vi "ReadWrite.vi"(8 "error in (no error)":errorcluster, 11 "Node Ptr":T2 format="%.0x") -> (0 "error out":errorcluster)   [LabVIEW 2017, in "Shared Variables CD 2.0 Configuration.lvlib"]
uses:
  Shared Variables CD 2.0 Configuration.lvlib
  <vilib>/NI Veristand/Custom Device API/Custom Device Item Ref.ctl
  Support/Add SV Process/Channel Configuration States.ctl
  Support/ChannelVS/ChannelVS.lvclass
  C:/Users/Public/Documents/National Instruments/NI VeriStand 2017/Custom Devices/Shared Variables CD 2.0/Data/Channel.lvlibp/Channel.lvclass
  <vilib>/Utility/VariantDataType/Type.ctl
  Support/ChannelVS/ChannelVS.lvclass/ChannelVS.ctl
  Support/ChannelVS/Compare Ch with Ch List.vi
  Support/ChannelVS/Read VeriSTAND Channel Info.vi
  Support/ChannelVS/Write VeriSTAND Channel Info.vi
  Shared/SV Global.vi
  Public/Documents/National Instruments/NI VeriStand 2017/Custom Devices/Shared Variables CD 2.0/Data/Channel.lvlibp/Read Channel Info.vi
  <vilib>/NI VeriStand/Custom Device API/Custom Device API.lvlib
  <vilib>/Utility/VariantDataType/VariantType.lvlib
panel:
  out "State":T1
  in  "Remove Button":bool
  in  "Add Button":bool
  in  "Refresh Target":bool
  in  "Target IPAddr":string caption="Target IP Address*"
  in  "Target List":string[](tree)
  in  "CD List":string[](tree)
  in  "Header":cluster{"Section Name":string}={"Section Name"="Custom Device Item Settings"}
  in  "Description":string
  in  "Name":string
  # "*Do Not Use \"localhost\" or host name"
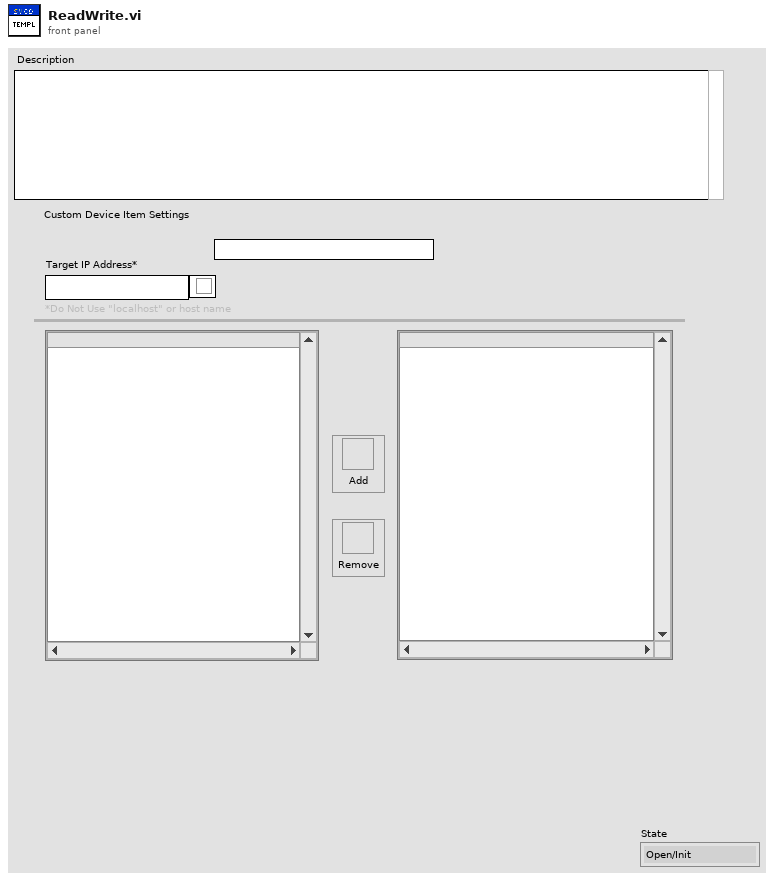
[diagram p1: front panel]
types:
  T1 = typedef "Shared Variables CD 2.0 Configuration.lvlib/Channel Configuration States.ctl" = enum16{"Open/Init", "Start Update", "Get VS Channels", "Get Available Ch from Target", "Wait On User Action", "Update Target Tree", "Update VS Trees", "Update Done", "Create VS Channels", "Remove VS Channels", "Error", "Close"}
  T2 = typedef "Custom Device API.lvlib/Custom Device Item Ref.ctl" = u64
  T3 = cluster{"Read Channel Array":refnum<class "ChannelVS.lvclass">[], "Write Channel Array":refnum<class "ChannelVS.lvclass">[]}
  T4 = enum8{"Enabled", "Disabled", "Disabled and Grayed Out"}
  T5 = typedef "VariantType.lvlib/Type.ctl" = enum8{"Invalid Type", "Void", "I8", "I16", "I32", "I64", "U8", "U16", "U32", "U64", "Single Float", "Double Float", "Extended Float", "Single Complex", "Double Complex", "Extended Complex", "Enum U8", "Enum U16", "Enum U32", "Enum U64", "Single Float With Unit", "Double Float With Unit", "Extended Float With Unit", "Single Complex with Unit", "Double Complex with Unit", "Extended Complex with Unit", "Boolean", "String", "Path", "Picture", "Tag", "Array", "Cluster", "Variant", "LV Variant", "Waveform", "Timestamp", "Digital Waveform", "Digital Data", "ExpressData", "Refnum", "External Data", "VI", "Poly VI", "LabVIEW Class Instance", "Fixed Point"}
  T6 = typedef "Custom Device API.lvlib/Custom Device Item Info.ctl" = cluster{"Name":string, "Is Channel":bool, "GUID":string, "Is Waveform":bool}
  T7 = typedef "Custom Device API.lvlib/Custom Device Commands.ctl" = enum16{"Default", "Item renamed", "Shutdown", "Dynamic button pressed"}
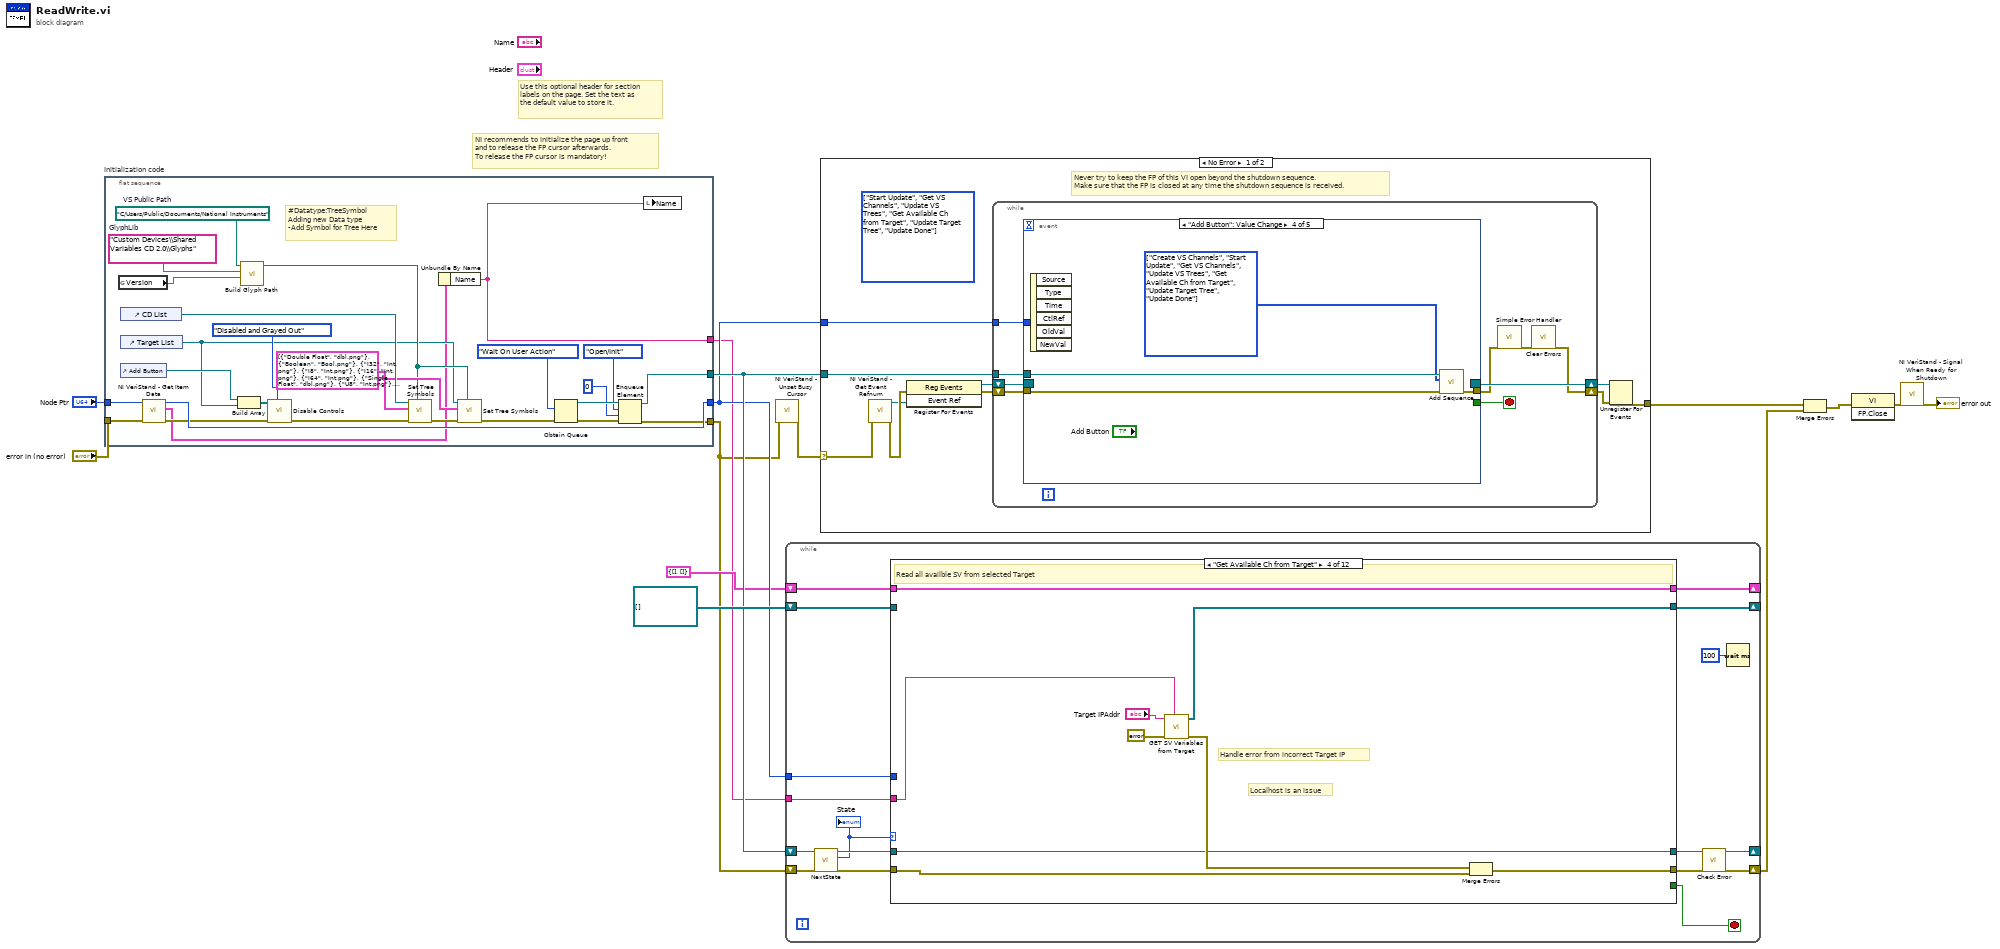
[diagram p0: block diagram]
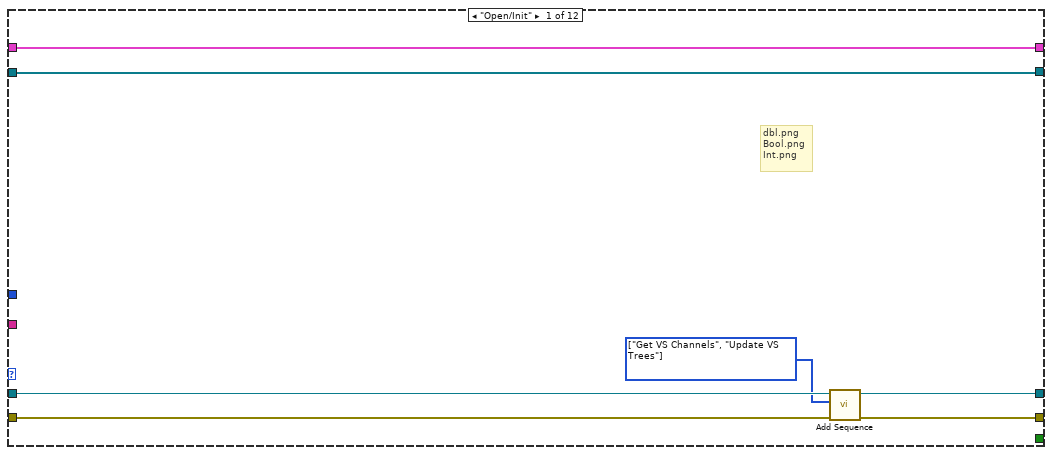
[diagram p2: hidden frame]
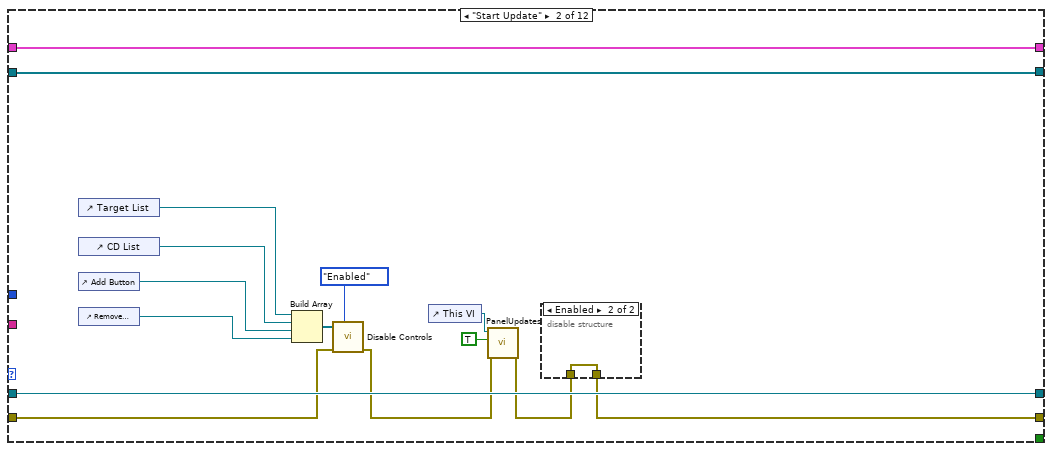
[diagram p3: hidden frame]
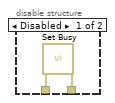
[diagram p4: hidden frame]
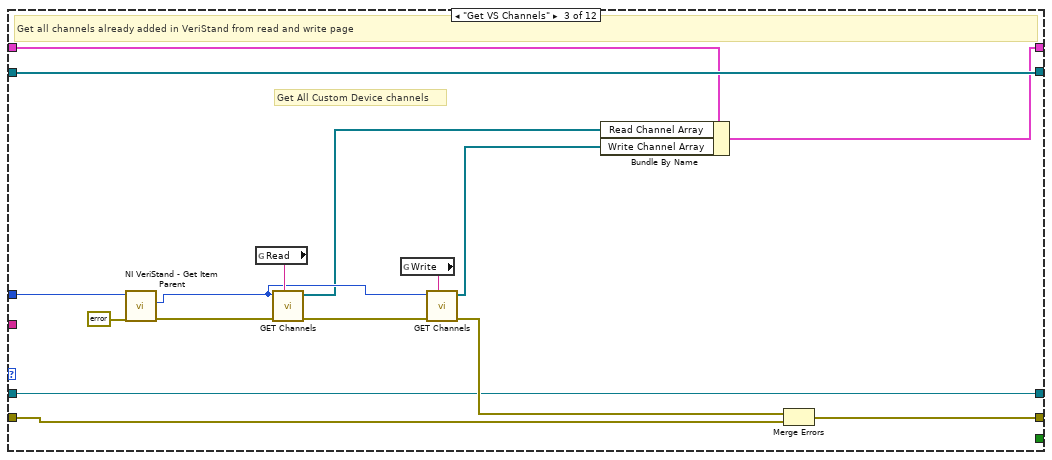
[diagram p5: hidden frame]
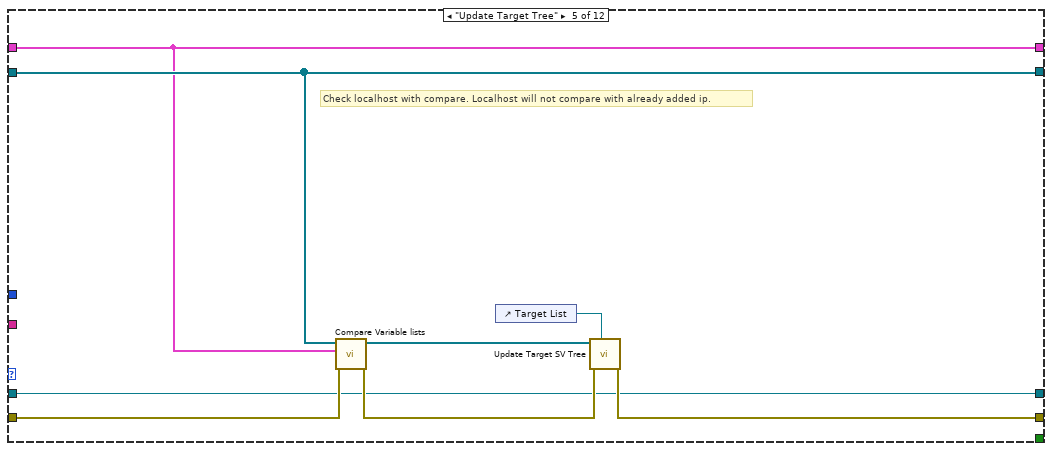
[diagram p6: hidden frame]
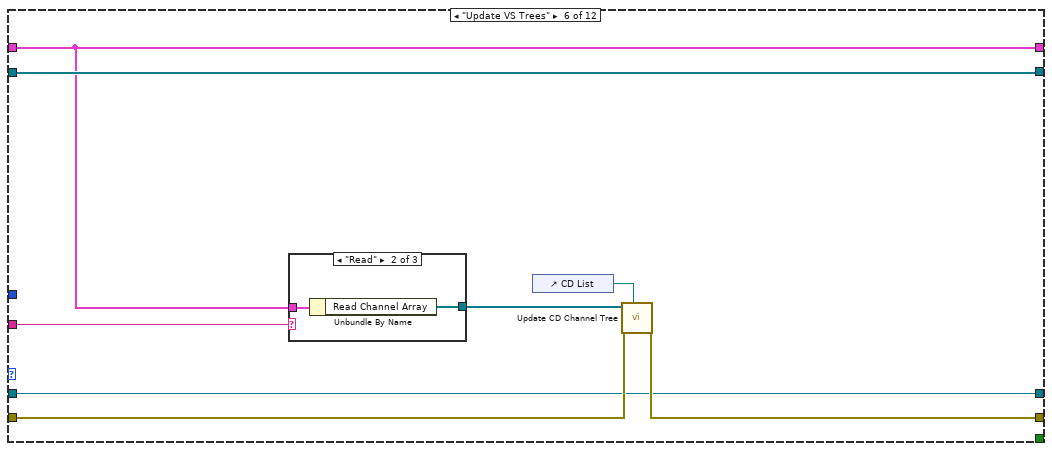
[diagram p7: hidden frame]
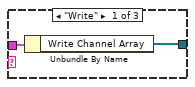
[diagram p8: hidden frame]
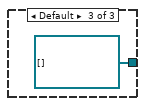
[diagram p9: hidden frame]
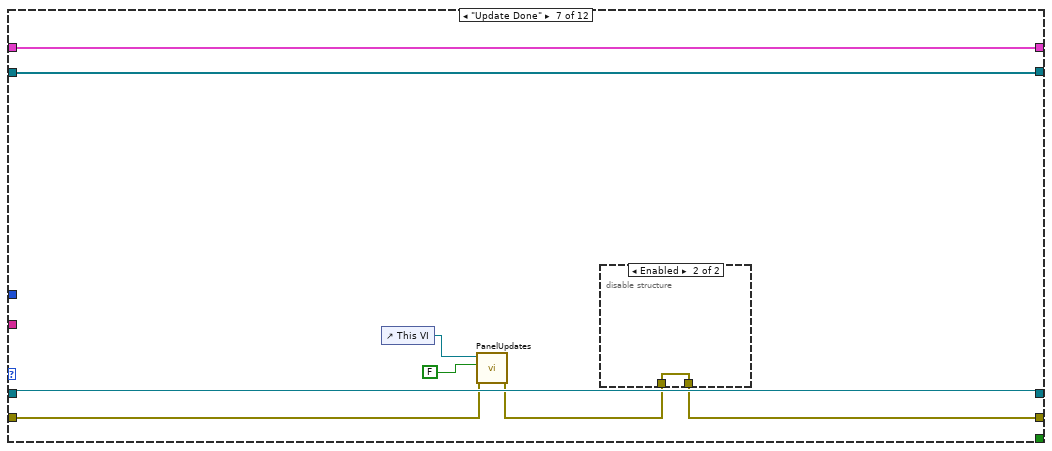
[diagram p10: hidden frame]
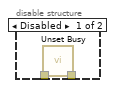
[diagram p11: hidden frame]
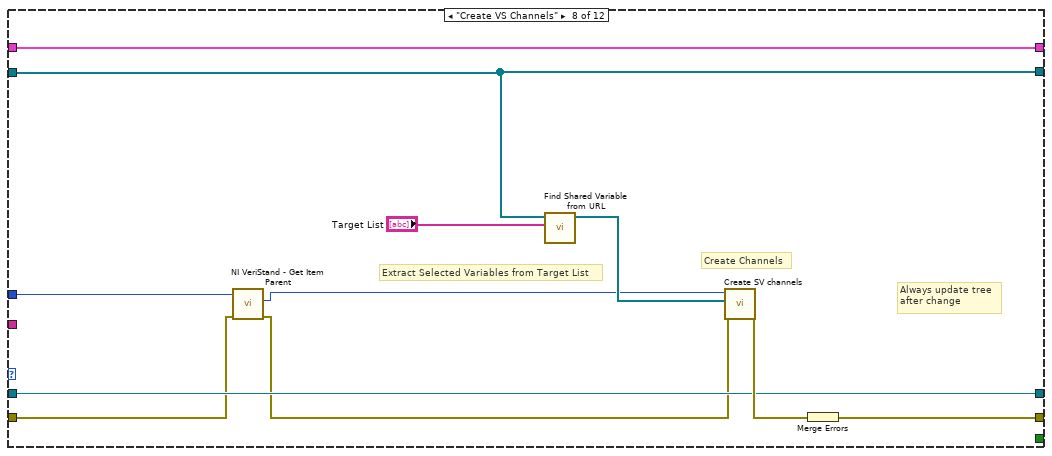
[diagram p12: hidden frame]
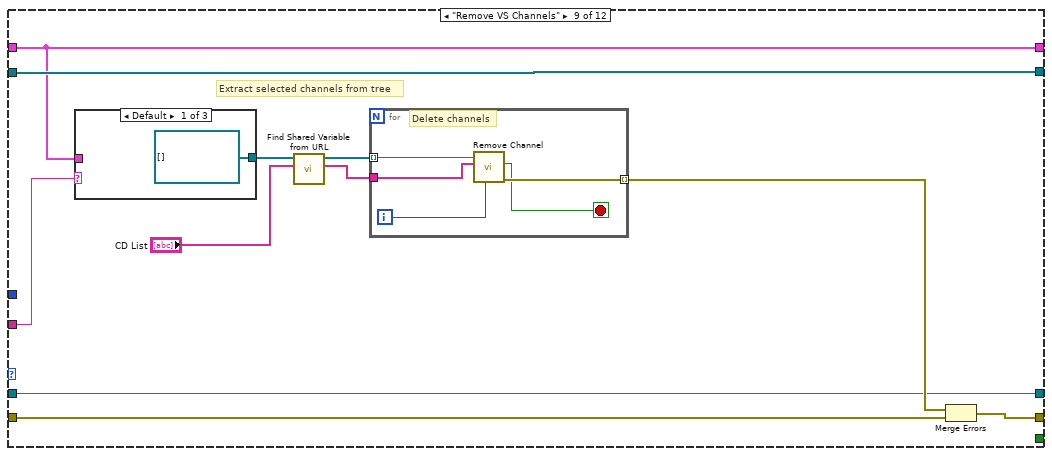
[diagram p13: hidden frame]
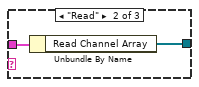
[diagram p14: hidden frame]
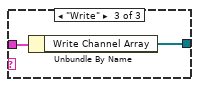
[diagram p15: hidden frame]
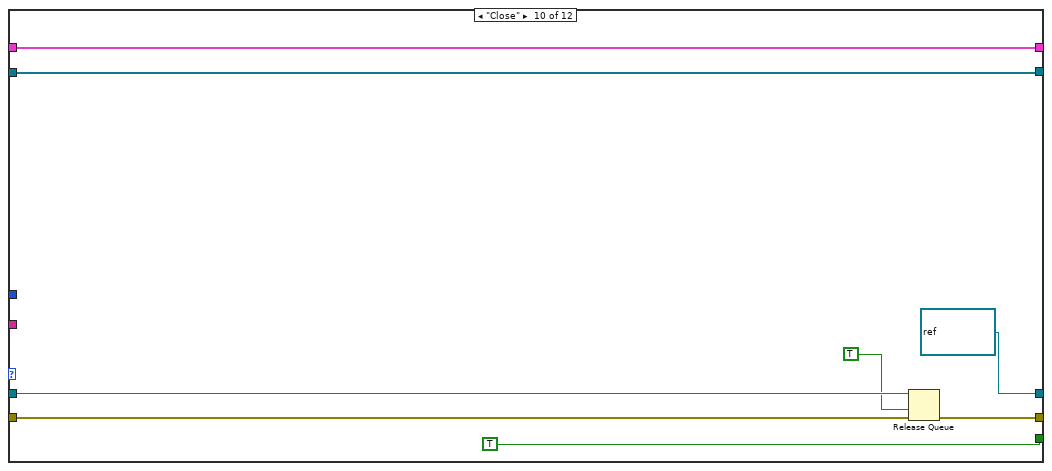
[diagram p16: hidden frame]
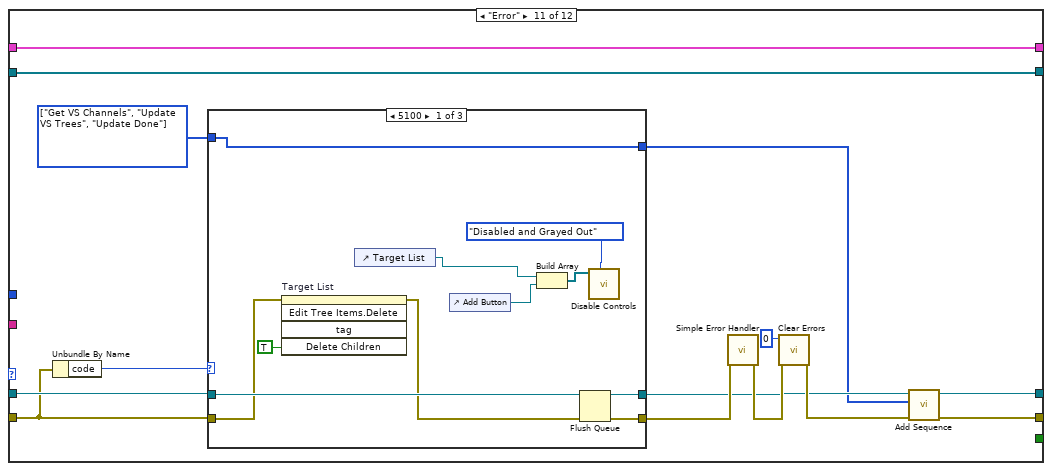
[diagram p17: hidden frame]
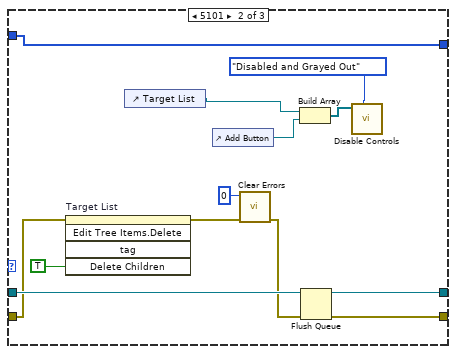
[diagram p18: hidden frame]
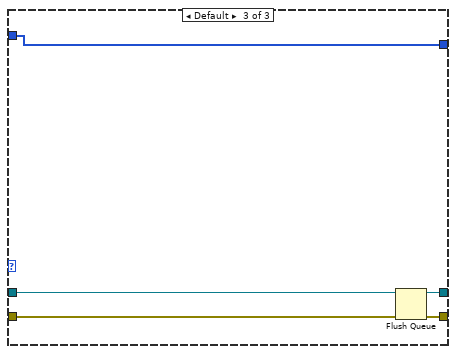
[diagram p19: hidden frame]
diagram:
  # "Use this optional header for section labels on the page. Set the text as the default value to store it."
  # "NI recommends to initialize the page up front\nand to release the FP cursor afterwards.\nTo release the FP cursor is mandatory!"
  n1 = flat-sequence "Initialization code" {
    tunnel: "error in (no error)" -> [w38]
    tunnel: "Node Ptr" -> [w39]
    tunnel: [w40] -> w6
    tunnel: [w25] -> w1
    tunnel: [w24] -> w7
    tunnel: [w15] -> w4
    frame #0 {
      w36 = path "C:/Users/Public/Documents/National Instruments"  # VS Public Path
      w37 = "Custom Devices\\Shared Variables CD 2.0\\Glyphs"  # GlyphLib
      w32 = cluster{"Type":T5, string}[] [{"Type"=enum."Double Float", "dbl.png"}, {"Type"=enum."Boolean", "Bool.png"}, {"Type"=enum."I32", "Int.png"}, {"Type"=enum."I8", "Int.png"}, {"Type"=enum."I16", "Int.png"}, {"Type"=enum."I64", "Int.png"}, {"Type"=enum."Single Float", "dbl.png"}, {"Type"=enum."U8", "Int.png"}, {"Type"=enum."U16", "Int.png"}, {"Type"=enum."U32", "Int.png"}, {"Type"=enum."U64", "Int.png"}]
      # "#Datatype:TreeSymbol\nAdding new Data type\n-Add Symbol for Tree Here"
      n2 = global read "SV Global.vi" "Version"() -> (w35:string)
      n3 = control-ref of="CD List"() -> (w34:refnum<vi>)
      n4 = control-ref of="Add Button"() -> (w22:refnum<vi>)
      n5 = control-ref of="Target List"() -> (w18:refnum<vi>)
      n6 = call <vilib>:"NI VeriStand - Get Item Data.vi"("error in (no error)"=w38, "Item Ref in"=w39) -> ("error out"=w20:errorcluster, "Item Info"=w16:T6, "Item Ref out"=w40:T2)  [unwired: 6 in, 1 out]
      n7 = Build Array(w22, w18) -> (w23:refnum<vi>[])
      n8 = call "Build Glyph Path.vi"("Version"=w35, "GlyphLib"=w37, "VS Public Path"=w36) -> ("Path to Glyph Lib"=w31:path)  [unwired: 8 in]
      n9 = call "Disable Controls.vi"("Disabled"=T4."Disabled and Grayed Out", "error in (no error)"=w20, "Array"=w23) -> ("error out"=w19:errorcluster)  [unwired: 8 in]
      n10 = call "Set Tree Symbols.vi"("Path to PNG lib"=w31, "error in (no error)"=w19, "Index and Image"=w32, "TreeControl in"=w34) -> ("error out"=w33:errorcluster)  [unwired: 7 in]
      n11 = Unbundle By Name(w16) -> ("Name"=w15:string)
      n12 = call "Set Tree Symbols.vi"("Path to PNG lib"=w31, "error in (no error)"=w33, "Index and Image"=w32, "TreeControl in"=w18) -> ("error out"=w17:errorcluster)  [unwired: 7 in]
      n13 = Obtain Queue(element data type=Channel_Configuration_States."Wait On User Action", error in (no error)=w17) -> (queue out=w30:refnum<queue>, error out=w29:errorcluster)  [unwired: 3 in, 1 out]
      n14 = Enqueue Element(queue=w30, element=Channel_Configuration_States."Open/Init", timeout in ms (-1)=0, error in (no error)=w29) -> (queue out=w24:refnum<queue>, error out=w25:errorcluster)  [unwired: 1 out]
      n15 = local write "Name"(w15) -> ()
    }
  }
  n16 = call <vilib>:"NI VeriStand - Unset Busy Cursor.vi"("error in (no error)"=w1) -> ("error out"=w10:errorcluster)  [unwired: 10 out]
  n17 = while {
    shift-right: [w50] -> w2
    shift-left: w1 -> [w43]
    shift-right: [w57] -> _
    shift-left: T3 {"Read Channel Array"=[], "Write Channel Array"=[]} -> [w56]
    shift-right: [w54] -> _
    shift-left: refnum<class "ChannelVS.lvclass">[] [] ("Channel Array") -> [w53]
    shift-right: [w45] -> _
    shift-left: w7 -> [w49]
    tunnel: w6 -> [w42]
    tunnel: w4 -> [w41]
    stop <- w55 stop-if-true
    n18 = call "NextState.vi"("error in (no error)"=w43, "Queue in"=w49) -> ("error out"=w44:errorcluster, "Next State"=w47:T1, "Queue out"=w48:refnum<queue>)  [unwired: 7 in]
    "State" <- w47
    n19 = case shown="\"Get Available Ch from Target\"" w47 {
      tunnel: w44 -> [w58 w67 w95 w103 w113 w121 w133 w145 w161 w176 w189 w226]
      tunnel: [w60 w68 w96 w104 w115 w120 w129 w148 w158 w175 w183 w226] -> w51
      tunnel: [w64 w79 w84 w107 w109 w122 w136 w150 w159 w178 w193 w225] -> w57
      tunnel: w56 -> [w64 w79 w83 w107 w109 w122 w136 w150 w159 w178 w193 w225]
      tunnel: [_ _ _ _ _ _ _ _ _ TRUE _ _] -> w55
      tunnel: [w63 w78 w98 w101 w111 w123 w135 w142 w160 w177 w192 w224] -> w54
      tunnel: w53 -> [w63 w78 w98 _ w111 w123 w135 w142 w160 w177 w192 w224]
      tunnel: w48 -> [w62 w72 w93 w102 w112 w119 w134 w147 w156 w174 w190 w223]
      tunnel: [w61 w72 w93 w102 w112 w119 w134 w147 w156 w172 w181 w223] -> w46
      tunnel: w42 -> [_ _ w85 _ _ _ _ w140 _ _ _ _]
      tunnel: w41 -> [_ _ _ w99 _ w116 _ _ w151 _ _ _]
      frame "Open/Init" {
        w59 = T1[] [enum."Get VS Channels", enum."Update VS Trees"] items=["Open/Init", "Start Update", "Get VS Channels", "Get Available Ch from Target", "Wait On User Action", "Update Target Tree", "Update VS Trees", "Update Done", "Create VS Channels", "Remove VS Channels", "Error", "Close"]
        # "dbl.png\nBool.png\nInt.png"
        n20 = call "Add Sequence.vi"("error in (no error)"=w58, "Transition Sequence"=w59, "Queue in"=w62) -> ("error out"=w60:errorcluster, "Queue out"=w61:refnum<queue>)  [unwired: 7 in]
      }
      frame "Start Update" {
        n21 = control-ref of="Target List"() -> (w65:refnum<vi>)
        n22 = control-ref of="CD List"() -> (w76:refnum<vi>)
        n23 = control-ref of="Add Button"() -> (w77:refnum<vi>)
        n24 = control-ref of="Remove Button"() -> (w74:refnum<vi>)
        n25 = Build Array(w65, w76, w77, w74) -> (w73:refnum<vi>[])
        n26 = call "Disable Controls.vi"("Disabled"=T4."Enabled", "error in (no error)"=w67, "Array"=w73) -> ("error out"=w66:errorcluster)  [unwired: 8 in]
        n27 = control-ref of="This VI"() -> (w70:refnum<vi>)
        n28 = call "PanelUpdates.vi"("error in (no error)"=w66, "Defer Panel Updates"=TRUE, "VI in"=w70) -> ("error out"=w69:errorcluster)  [unwired: 8 in]
        n29 = disable-structure shown="Enabled" {
          disable-tunnel: w69 -> [w81 w82]
          disable-tunnel: [w80 w82] -> w68
          frame Disabled {
            n30 = call <vilib>:"Set Busy.vi"("error in (no error)"=w81) -> ("error out"=w80:errorcluster)  [unwired: 9 in, 1 out]
          }
          frame Enabled {
          }
        }
      }
      frame "Get VS Channels" {
        # "Get All Custom Device channels"
        # "Get all channels already added in VeriStand from read and write page"
        n31 = call <vilib>:"NI VeriStand - Get Item Parent.vi"("error in (no error)"=errorcluster {"status"=FALSE, "code"=0, "source"=""}, "Item Ref in"=w85) -> ("error out"=w90:errorcluster, "Parent Ref"=w88:T2)  [unwired: 6 in, 2 out]
        n32 = global read "SV Global.vi" "Read"() -> (w91:string)
        n33 = call "GET Channels.vi"("Channel Direction"=w91, "error in (no error)"=w90, "Item Ref in"=w88) -> ("error out"=w89:errorcluster, "VS Channel Array"=w87:refnum<class "ChannelVS.lvclass">[])  [unwired: 7 in]
        n34 = global read "SV Global.vi" "Write"() -> (w92:string)
        n35 = call "GET Channels.vi"("Channel Direction"=w92, "error in (no error)"=w89, "Item Ref in"=w88) -> ("error out"=w97:errorcluster, "VS Channel Array"=w86:refnum<class "ChannelVS.lvclass">[])  [unwired: 7 in]
        n36 = Bundle By Name(cluster=w83, "Read Channel Array"=w87, "Write Channel Array"=w86) -> (w84:T3)
        n37 = Merge Errors(w97, w95) -> (w96:errorcluster)
      }
      frame "Get Available Ch from Target" {
        # "Localhost is an issue"
        # "Handle error from incorrect Target IP"
        # "Read all availble SV from selected Target"
        n38 = call "GET SV Variables from Target.vi"("Read/Write"=w99, "error in (no error)"=errorcluster {"status"=FALSE, "code"=0, "source"=""}, "Target"="Target IPAddr") -> ("error out"=w106:errorcluster, "Channel Array"=w101:refnum<class "ChannelVS.lvclass">[])  [unwired: 7 in]
        n39 = Merge Errors(w106, w103) -> (w104:errorcluster)
      }
      frame "Update Target Tree" {
        # "Check localhost with compare. Localhost will not compare with already added ip."
        n40 = call "Compare Variable lists.vi"("error in (no error)"=w113, "Channel Arrays"=w109, "Variable List"=w111) -> ("error out"=w114:errorcluster, "Variable list compared"=w110:refnum<class "ChannelVS.lvclass">[])  [unwired: 7 in]
        n41 = control-ref of="Target List"() -> (w108:refnum<vi>)
        n42 = call "Update Target SV Tree.vi"("TreeControl in"=w108, "error in (no error)"=w114, "Variable list compared"=w110) -> ("error out"=w115:errorcluster)  [unwired: 8 in]
      }
      frame "Update VS Trees" {
        n43 = case shown="\"Read\"" w116 {
          tunnel: [w125 w127 refnum<class "ChannelVS.lvclass">[] [] ("Read Channel Array")] -> w118
          tunnel: w122 -> [w124 w126 _]
          frame "Write" {
            n44 = Unbundle By Name(w124) -> ("Write Channel Array"=w125:refnum<class "ChannelVS.lvclass">[])
          }
          frame "Read" {
            n45 = Unbundle By Name(w126) -> ("Read Channel Array"=w127:refnum<class "ChannelVS.lvclass">[])
          }
          frame Default {
          }
        }
        n46 = control-ref of="CD List"() -> (w117:refnum<vi>)
        n47 = call "Update CD Channel Tree.vi"("CD List"=w117, "error in (no error)"=w121, "Channel Array"=w118) -> ("error out"=w120:errorcluster)  [unwired: 8 in]
      }
      frame "Update Done" {
        n48 = control-ref of="This VI"() -> (w132:refnum<vi>)
        n49 = call "PanelUpdates.vi"("error in (no error)"=w133, "Defer Panel Updates"=FALSE, "VI in"=w132) -> ("error out"=w130:errorcluster)  [unwired: 8 in]
        n50 = disable-structure shown="Enabled" {
          disable-tunnel: w130 -> [w138 w139]
          disable-tunnel: [w137 w139] -> w129
          frame Disabled {
            n51 = call <vilib>:"Unset Busy.vi"("error in (no error)"=w138) -> ("error out"=w137:errorcluster)  [unwired: 10 in]
          }
          frame Enabled {
          }
        }
      }
      frame "Create VS Channels" {
        # "Create Channels"
        # "Extract Selected Variables from Target List"
        # "Always update tree\nafter change"
        n52 = call <vilib>:"NI VeriStand - Get Item Parent.vi"("error in (no error)"=w145, "Item Ref in"=w140) -> ("error out"=w144:errorcluster, "Parent Ref"=w143:T2)  [unwired: 6 in, 2 out]
        n53 = call "Find Shared Variable from URL.vi"("Target List"="Target List", "Variable List"=w142) -> ("Variable info"=w146:refnum<class "ChannelVS.lvclass">[])  [unwired: 8 in, 1 out]
        n54 = call "Create SV channels.vi"("error in"=w144, "Variable List"=w146, "Custom Device in"=w143) -> ("error out"=w149:errorcluster)  [unwired: 7 in, 1 out]
        n55 = Merge Errors(w149) -> (w148:errorcluster)
      }
      frame "Remove VS Channels" {
        # "Extract selected channels from tree"
        n56 = case shown="Default" w151 {
          tunnel: w159 -> [_ w168 w171]
          tunnel: [refnum<class "ChannelVS.lvclass">[] [] ("Write Channel Array") w169 w170] -> w154
          frame Default {
          }
          frame "Read" {
            n57 = Unbundle By Name(w168) -> ("Read Channel Array"=w169:refnum<class "ChannelVS.lvclass">[])
          }
          frame "Write" {
            n58 = Unbundle By Name(w171) -> ("Write Channel Array"=w170:refnum<class "ChannelVS.lvclass">[])
          }
        }
        n59 = call "Find Shared Variable from URL.vi"("Target List"="CD List", "Variable List"=w154) -> ("Sort Name List"=w155:string[], "Variable info"=w153:refnum<class "ChannelVS.lvclass">[])  [unwired: 8 in]
        n60 = for {
          tunnel: [w166] -> w157 mode=indexing
          tunnel: w155 -> [w164]
          tunnel: w153 -> [w162] mode=indexing
          i -> [w165]
          stop <- w163 stop-if-true
          # "Delete channels"
          n61 = call "Remove Channel.vi"("Index from Loop Node (0)"=w165, "Name List"=w164, "ChannelVS in"=w162) -> ("error out"=w166:errorcluster, "Cancelled"=w163:bool)  [unwired: 7 in]
        }
        n62 = Merge Errors(w157, w161) -> (w158:errorcluster)
      }
      frame "Close" {
        w172 = refnum<queue> refnum items=["Open/Init", "Start Update", "Get VS Channels", "Get Available Ch from Target", "Wait On User Action", "Update Target Tree", "Update VS Trees", "Update Done", "Create VS Channels", "Remove VS Channels", "Error", "Close"] ("queue out")
        n63 = Release Queue(queue=w174, force destroy? (F)=TRUE, error in (no error)=w176) -> (error out=w175:errorcluster)  [unwired: 2 out]
      }
      frame "Error" {
        w187 = T1[] [enum."Get VS Channels", enum."Update VS Trees", enum."Update Done"] items=["Open/Init", "Start Update", "Get VS Channels", "Get Available Ch from Target", "Wait On User Action", "Update Target Tree", "Update VS Trees", "Update Done", "Create VS Channels", "Remove VS Channels", "Error", "Close"]
        n64 = Unbundle By Name(w189) -> ("code"=w188:i32)
        n65 = case shown="5100" w188 {
          tunnel: [w201 w214 w222] -> w182
          tunnel: [w200 w213 w221] -> w186
          tunnel: w190 -> [w199 w212 w220]
          tunnel: w189 -> [w197 w208 w219]
          tunnel: [w198 w209 w218] -> w180
          tunnel: w187 -> [w198 w209 w218]
          frame 5100 {
            n66 = invoke on="Target List" class="Tree (strict)" method="Edit Tree Items.Delete"(error in=w197, "Delete Children"=TRUE ("Delete Children?")) -> (error out=w196:errorcluster)  [unwired: 3 in, 4 out]
            n67 = control-ref of="Target List"() -> (w194:refnum<vi>)
            n68 = control-ref of="Add Button"() -> (w203:refnum<vi>)
            n69 = Build Array(w194, w203) -> (w202:refnum<vi>[])
            n70 = Flush Queue(queue=w199, error in (no error)=w196) -> (queue out=w201:refnum<queue>, error out=w200:errorcluster)  [unwired: 1 out]
            n71 = call "Disable Controls.vi"("Disabled"=T4."Disabled and Grayed Out", "Array"=w202) -> ()  [unwired: 9 in, 1 out]
          }
          frame 5101 {
            n72 = invoke on="Target List" class="Tree (strict)" method="Edit Tree Items.Delete"(error in=w208, "Delete Children"=TRUE ("Delete Children?")) -> (error out=w207:errorcluster)  [unwired: 3 in, 4 out]
            n73 = control-ref of="Target List"() -> (w205:refnum<vi>)
            n74 = control-ref of="Add Button"() -> (w216:refnum<vi>)
            n75 = call <vilib>:"Clear Errors.vi"("error in (no error)"=w207, "specific error code to clear (0: all)"=0) -> ("error out"=w211:errorcluster)  [unwired: 4 in, 1 out]
            n76 = Build Array(w205, w216) -> (w215:refnum<vi>[])
            n77 = Flush Queue(queue=w212, error in (no error)=w211) -> (queue out=w214:refnum<queue>, error out=w213:errorcluster)  [unwired: 1 out]
            n78 = call "Disable Controls.vi"("Disabled"=T4."Disabled and Grayed Out", "Array"=w215) -> ()  [unwired: 9 in, 1 out]
          }
          frame Default {
            n79 = Flush Queue(queue=w220, error in (no error)=w219) -> (queue out=w222:refnum<queue>, error out=w221:errorcluster)  [unwired: 1 out]
          }
        }
        n80 = call <vilib>:"Simple Error Handler.vi"("error in (no error)"=w186) -> ("error out"=w191:errorcluster)  [unwired: 4 in, 4 out]
        n81 = call <vilib>:"Clear Errors.vi"("error in (no error)"=w191, "specific error code to clear (0: all)"=0) -> ("error out"=w184:errorcluster)  [unwired: 4 in, 1 out]
        n82 = call "Add Sequence.vi"("error in (no error)"=w184, "Transition Sequence"=w180, "Queue in"=w182) -> ("error out"=w183:errorcluster, "Queue out"=w181:refnum<queue>)  [unwired: 7 in]
      }
      frame Default {
      }
    }
    n83 = call "Check Error.vi"("error in (no error)"=w51, "queue in"=w46) -> ("error out"=w50:errorcluster, "queue out"=w45:refnum<queue>)  [unwired: 8 in]
    n84 = Wait (ms)(milliseconds to wait=u32 100) -> ()  [unwired: 1 out]
  }
  n85 = case shown="No Error" w10 {
    selector: w10 -> [w228 w288]
    tunnel: [w233 w286] -> w14
    tunnel: w6 -> [w229 _]
    tunnel: w7 -> [w227 _]
    frame No Error {
      (unwired) T1[] [enum."Start Update", enum."Get VS Channels", enum."Update VS Trees", enum."Get Available Ch from Target", enum."Update Target Tree", enum."Update Done"] items=["Open/Init", "Start Update", "Get VS Channels", "Get Available Ch from Target", "Wait On User Action", "Update Target Tree", "Update VS Trees", "Update Done", "Create VS Channels", "Remove VS Channels", "Error", "Close"]
      # "Never try to keep the FP of this VI open beyond the shutdown sequence.\nMake sure that the FP is closed at any time the shutdown sequence is received."
      n86 = call <vilib>:"NI VeriStand - Get Event Refnum.vi"("error in (no error)"=w228) -> ("error out"=w236:errorcluster, "Event Ref"=w232:refnum<user-event>)  [unwired: 9 out]
      n87 = register-events(error in=w236, w232) -> (reference out=w230:refnum<event-registration>, error out=w231:errorcluster)  [unwired: 1 in]
      n88 = while {
        tunnel: w229 -> [w241]
        shift-right: [w238] -> w234
        shift-left: w231 -> [w244]
        shift-right: [w245] -> w235
        shift-left: w230 -> [w243]
        tunnel: w227 -> [w237]
        stop <- w242 stop-if-true
        n89 = event shown="[3] \"Add Button\": Value Change" {
          selector: w243 -> [_ _ _ _ _]
          dyn-events: [_ _ _ _ _] -> w245
          timeout: _ -> [_ _ _ _ _]
          tunnel: w244 -> [w254 w272 w276 w280 w284]
          tunnel: [w250 _ _ _ _] -> w242
          tunnel: [w249 w271 w275 w279 w283] -> w240
          tunnel: w241 -> [w248 w273 _ _ _]
          tunnel: w237 -> [w246 _ w277 w281 w285]
          event User Event {
            n90 = event-data() -> ("Data"=w253:string)  [unwired: 1 out]
            n91 = call <vilib>:"NI VeriStand - Parse Incoming Command Data.vi"("error in (no error)"=w254, "Incoming data"=w253) -> ("error out"=w252:errorcluster, "Outgoing data"=w247:variant, "Action"=w251:T7)  [unwired: 7 out]
            n92 = case shown="\"Shutdown\"" w251 {
              tunnel: w252 -> [w255 w260 w263 w269]
              tunnel: [_ _ TRUE _] -> w250
              tunnel: [w255 w257 w262 w266] -> w249
              tunnel: w248 -> [_ w259 _ _]
              tunnel: w247 -> [_ _ _ w268]
              tunnel: w246 -> [_ _ w264 _]
              frame "Default", Default {
              }
              frame "Item renamed" {
                n93 = call <vilib>:"NI VeriStand - Get Item Data.vi"("error in (no error)"=w260, "Item Ref in"=w259) -> ("error out"=w257:errorcluster, "Item Info"=w258:T6)  [unwired: 8 out]
                n94 = Unbundle By Name(w258) -> ("Name"=w256:string)
                n95 = local write "Name"(w256) -> ()
              }
              frame "Shutdown" {
                w261 = T1[] [enum."Close"] items=["Open/Init", "Start Update", "Get VS Channels", "Get Available Ch from Target", "Wait On User Action", "Update Target Tree", "Update VS Trees", "Update Done", "Create VS Channels", "Remove VS Channels", "Error", "Close"] ("Transition Sequence")
                # "The page has received the command to save all its data and to acknowledge that the page is ready to get unloaded from memory."
                n96 = call "Add Sequence.vi"("error in (no error)"=w263, "Transition Sequence"=w261, "Queue in"=w264) -> ("error out"=w262:errorcluster)  [unwired: 7 in, 1 out]
              }
              frame "Dynamic button pressed" {
                w267 = ""  # Button ID
                # "The user has pressed one of the dynamic buttons"
                n97 = Variant To Data(error in=w269, type=w267, Variant=w268) -> (error out=w266:errorcluster)  [unwired: 1 out]
              }
            }
          }
          event "Description": Value Change {
            n98 = event-data() -> ()  [unwired: 2 out]
            n99 = call <vilib>:"NI VeriStand - Set Item Description.vi"("error in (no error)"=w272, "Description"="Description", "Item Ref in"=w273) -> ("error out"=w271:errorcluster)  [unwired: 8 out]
          }
          event "Refresh Target": Value Change {
            w274 = T1[] [enum."Start Update", enum."Get VS Channels", enum."Update VS Trees", enum."Get Available Ch from Target", enum."Update Target Tree", enum."Update Done"] items=["Open/Init", "Start Update", "Get VS Channels", "Get Available Ch from Target", "Wait On User Action", "Update Target Tree", "Update VS Trees", "Update Done", "Create VS Channels", "Remove VS Channels", "Error", "Close"]
            # "Standard Sequence for Update"
            n100 = event-data() -> ()  [unwired: 7 out]
            n101 = call "Add Sequence.vi"("error in (no error)"=w276, "Transition Sequence"=w274, "Queue in"=w277) -> ("error out"=w275:errorcluster)  [unwired: 7 in, 1 out]
          }
          event "Add Button": Value Change {
            w278 = T1[] [enum."Create VS Channels", enum."Start Update", enum."Get VS Channels", enum."Update VS Trees", enum."Get Available Ch from Target", enum."Update Target Tree", enum."Update Done"] items=["Open/Init", "Start Update", "Get VS Channels", "Get Available Ch from Target", "Wait On User Action", "Update Target Tree", "Update VS Trees", "Update Done", "Create VS Channels", "Remove VS Channels", "Error", "Close"]
            n102 = event-data() -> ()  [unwired: 7 out]
            n103 = call "Add Sequence.vi"("error in (no error)"=w280, "Transition Sequence"=w278, "Queue in"=w281) -> ("error out"=w279:errorcluster)  [unwired: 7 in, 1 out]
          }
          event "Remove Button": Value Change {
            w282 = T1[] [enum."Remove VS Channels", enum."Start Update", enum."Get VS Channels", enum."Update VS Trees", enum."Update Target Tree", enum."Update Done"] items=["Open/Init", "Start Update", "Get VS Channels", "Get Available Ch from Target", "Wait On User Action", "Update Target Tree", "Update VS Trees", "Update Done", "Create VS Channels", "Remove VS Channels", "Error", "Close"]
            n104 = event-data() -> ()  [unwired: 7 out]
            n105 = call "Add Sequence.vi"("error in (no error)"=w284, "Transition Sequence"=w282, "Queue in"=w285) -> ("error out"=w283:errorcluster)  [unwired: 7 in, 1 out]
          }
        }
        n106 = call <vilib>:"Simple Error Handler.vi"("error in (no error)"=w240) -> ("error out"=w239:errorcluster)  [unwired: 1 in, 7 out]
        n107 = call <vilib>:"Clear Errors.vi"("error in (no error)"=w239) -> ("error out"=w238:errorcluster)  [unwired: 1 in, 5 out]
      }
      n108 = Unregister For Events(event registration refnum=w235, error in=w234) -> (error out=w233:errorcluster)
    }
    frame Error {
      n109 = call <vilib>:"Simple Error Handler.vi"("error in (no error)"=w288) -> ("error out"=w287:errorcluster)  [unwired: 1 in, 7 out]
      n110 = call <vilib>:"Clear Errors.vi"("error in (no error)"=w287) -> ("error out"=w286:errorcluster)  [unwired: 1 in, 5 out]
    }
  }
  n111 = Merge Errors(w14, w2) -> (w3:errorcluster)
  n112 = invoke class="VI" method="FP.Close"(error in=w3) -> (error out=w13:errorcluster)  [unwired: 2 in, 2 out]
  n113 = call <vilib>:"NI VeriStand - Signal When Ready for Shutdown.vi"("error in (no error)"=w13) -> ("error out"=→"error out":errorcluster)  [unwired: 10 out]
